vi "Read _regionSet.vi"(8 "error in (no error)":errorcluster, 11 "HTTP Request in":refnum<class "HTTP Request.lvclass">) -> (0 "error out":errorcluster, 2 "_regionSet?":bool, 3 "HTTP Request out":refnum<class "HTTP Request.lvclass">)   [LabVIEW 2015, in "NI_AWS_Core.lvlib" / "HTTP Request.lvclass"]
uses:
  HTTP Request.lvclass
  HTTP Request.lvclass/HTTP Request.ctl
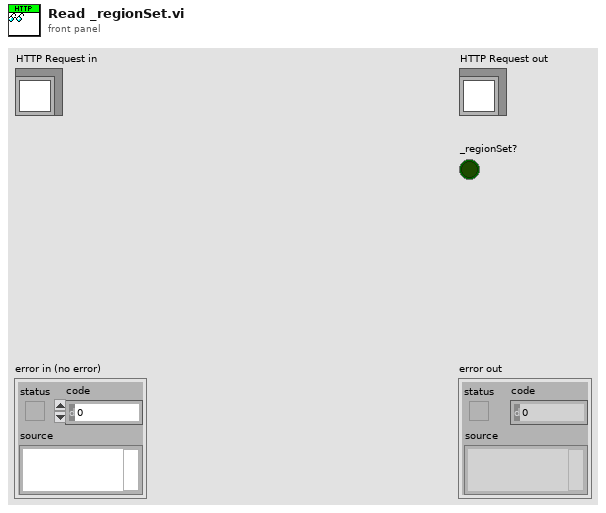
[diagram p1: front panel]
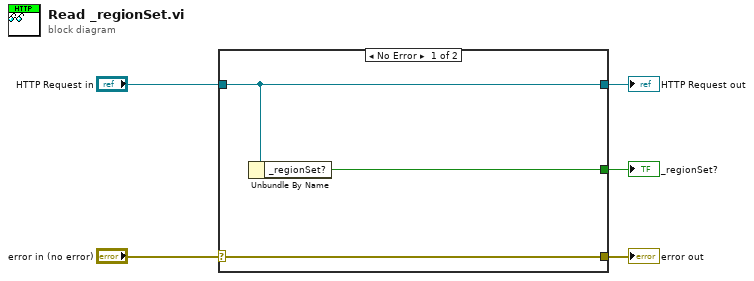
[diagram p0: block diagram]
diagram:
  n1 = case shown="No Error" "error in (no error)" {
    selector: "error in (no error)" -> [w8 w9]
    tunnel: [w8 w9] -> w4
    tunnel: [w7 w10] -> w2
    tunnel: "HTTP Request in" -> [w7 w10]
    tunnel: [w6 _] -> w1
    frame No Error {
      n2 = Unbundle By Name(w7) -> ("_regionSet?"=w6:bool)
    }
    frame Error {
    }
  }
  "error out" <- w4
  "HTTP Request out" <- w2
  "_regionSet?" <- w1
